vi "testCheckInputStringIsNotEmpty.vi"(8 "error in (no error)":errorcluster) -> (0 "error out":errorcluster)   [LabVIEW 2018]
doc: "Test checkInputStringIsNotEmpty.vi"
uses:
  src/TcpServerBase/TcpServerBase.lvclass
  src/TcpServerBase/TcpServerBase.lvclass/TcpServerBase.ctl
  <vilib>/addons/_JKI Toolkits/Caraya/classes/Assert/Assert Equal Value_Variant.vi
  <vilib>/addons/_JKI Toolkits/Caraya/classes/Test/Test.lvclass
  <vilib>/addons/_JKI Toolkits/Caraya/classes/Assert/Assert.lvclass
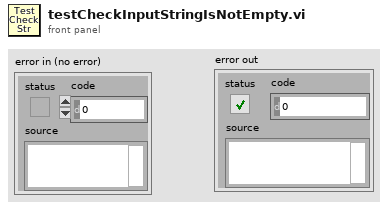
[diagram p1: front panel]
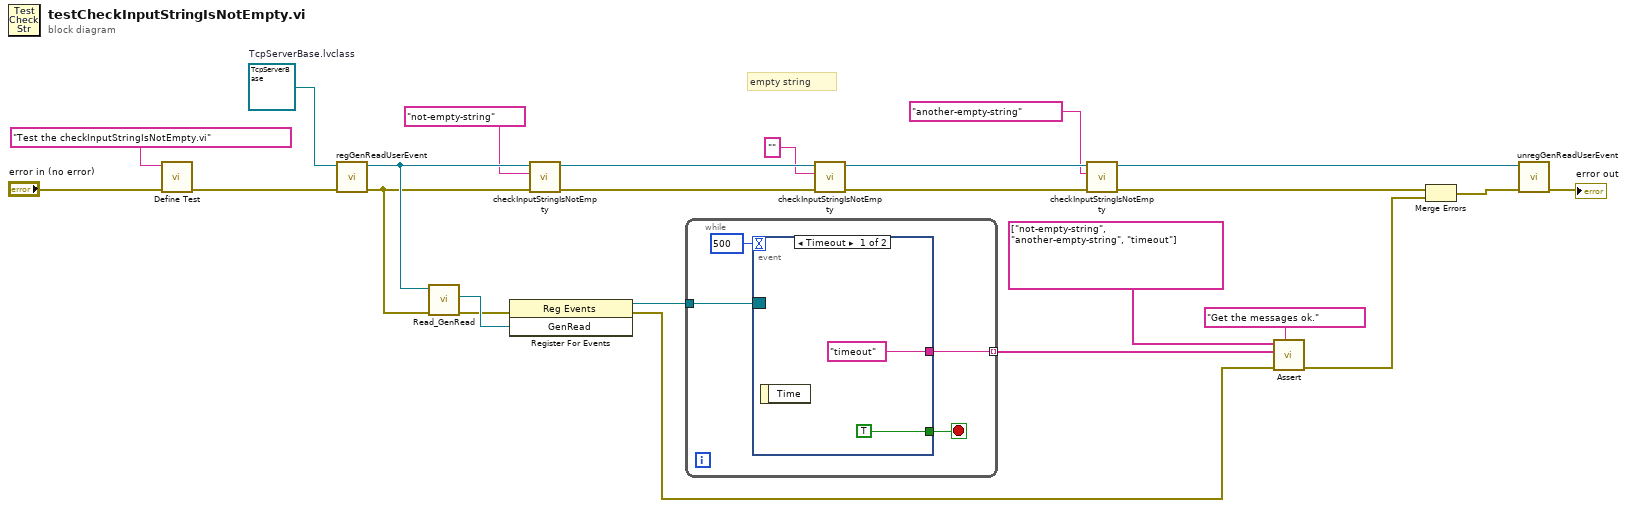
[diagram p0: block diagram]
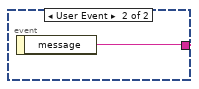
[diagram p2: hidden frame]
diagram:
  w20 = refnum<class "TcpServerBase.lvclass"> refnum  # TcpServerBase.lvclass
  # "empty string"
  n1 = call <vilib>:"Define Test.vi"("error in (no error)"="error in (no error)", "Label (VI Title)"="Test the checkInputStringIsNotEmpty.vi") -> ("error out"=w19:errorcluster)  [unwired: 9 in]
  n2 = call "regGenReadUserEvent.vi"("error in (no error)"=w19, "TcpServerBase in"=w20) -> ("error out"=w17:errorcluster, "TcpServerBase out"=w18:refnum<class "TcpServerBase.lvclass">)  [unwired: 8 in]
  n3 = call "Read_GenRead.vi"("error in (no error)"=w17, "TcpServerBase in"=w18) -> ("error out"=w21:errorcluster, "GenRead"=w22:refnum<user-event>)  [unwired: 7 in, 1 out]
  n4 = register-events(error in=w21, w22) -> (reference out=w15:refnum<event-registration>, error out=w8:errorcluster)  [unwired: 1 in]
  n5 = call "checkInputStringIsNotEmpty.vi"("error in (no error)"=w17, "inputString"="not-empty-string", "TcpServerBase in"=w18) -> ("error out"=w13:errorcluster, "TcpServerBase out"=w14:refnum<class "TcpServerBase.lvclass">)  [unwired: 7 in]
  n6 = while {
    tunnel: w15 -> [w29]
    tunnel: [w28] -> w6 mode=indexing
    stop <- w26 stop-if-true
    n7 = event shown="[0] Timeout" {
      selector: w29 -> [_ _]
      dyn-events: _ -> [_ _]
      timeout: 500 -> [_ _]
      tunnel: ["timeout" ("message") w32] -> w28
      tunnel: [TRUE _] -> w26
      event Timeout {
        n8 = event-data() -> ()  [unwired: 1 in, 1 out]
      }
      event User Event {
        n9 = event-data() -> ("message"=w32:string)  [unwired: 1 in]
      }
    }
  }
  n10 = call "checkInputStringIsNotEmpty.vi"("error in (no error)"=w13, "inputString"="", "TcpServerBase in"=w14) -> ("error out"=w10:errorcluster, "TcpServerBase out"=w11:refnum<class "TcpServerBase.lvclass">)  [unwired: 7 in]
  n11 = call "checkInputStringIsNotEmpty.vi"("error in (no error)"=w10, "inputString"="another-empty-string", "TcpServerBase in"=w11) -> ("error out"=w2:errorcluster, "TcpServerBase out"=w5:refnum<class "TcpServerBase.lvclass">)  [unwired: 7 in]
  n12 = call-poly <vilib>:"Assert.vi"("Label"="Get the messages ok.", "error in (no error)"=w8, "Y"=w6, "X"=string[] ["not-empty-string", "another-empty-string", "timeout"] ("message")) -> ("error out"=w4:errorcluster)  [unwired: 7 in]
  n13 = Merge Errors(w2, w4) -> (w3:errorcluster)
  n14 = call "unregGenReadUserEvent.vi"("error in (no error)"=w3, "tcpServerBase in"=w5) -> ("error out"=→"error out":errorcluster)  [unwired: 8 in, 1 out]
